vi "BS navigation demo.vi"() -> ()   [LabVIEW 2012]
uses:
  <vilib>/vision/NI_Vision_Development_Module.lvlib
panel:
  out "tug location string":string
  out "All found?":bool
  out "Tug location array":T1(array[cluster])
  in  "Image file name":string="boats and buoys.bmp"
  in  "stop":bool
  out "error out":errorcluster
  out "Working Image":T2(plugin-control)
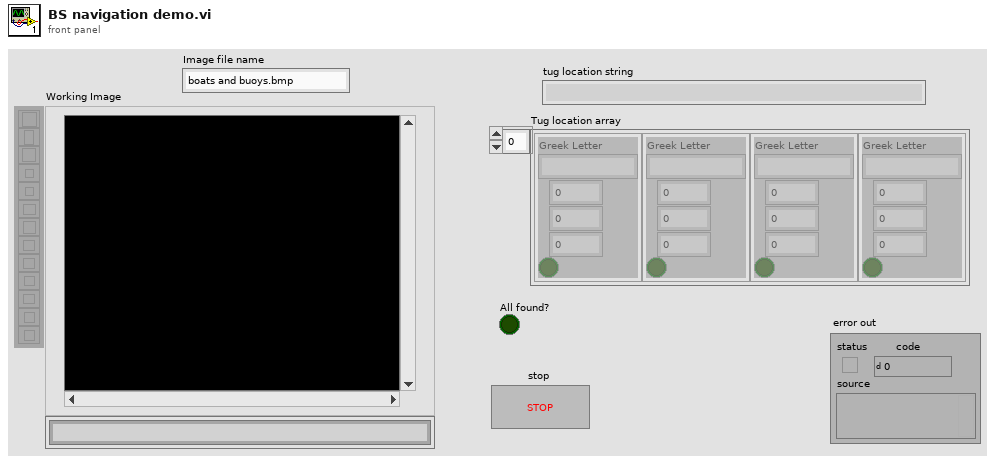
[diagram p1: front panel]
types:
  T1 = cluster{"Greek Letter":string, i16, i16, i16, bool}[]
  T2 = typedef "IMAQ Image.ctl" = refnum<image>
  T3 = typedef "Image Type" = u32
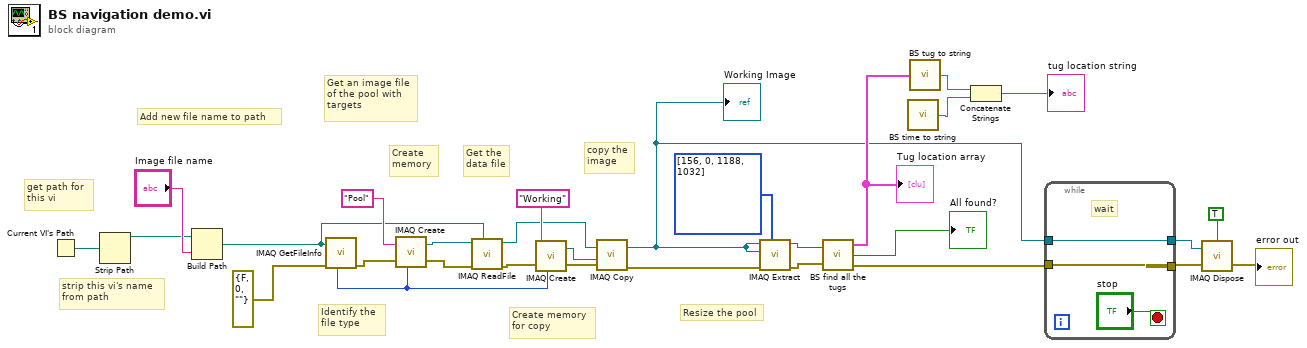
[diagram p0: block diagram]
diagram:
  # "Resize the pool"
  # "Create memory\nfor copy"
  # "copy the\nimage"
  # "Add new file name to path"
  # "strip this vi's name \nfrom path"
  # "get path for \nthis vi"
  # "Get the \ndata file"
  # "Create \nmemory"
  # "Identify the \nfile type"
  # "Get an image file\nof the pool with\ntargets"
  n1 = Current VI's Path() -> (path=w21:path)
  n2 = Strip Path(path=w21) -> (stripped path=w20:path)  [unwired: 1 out]
  n3 = Build Path(base path=w20, name or relative path="Image file name") -> (appended path=w19:path)
  n4 = call "IMAQ GetFileInfo"("error in (no error)"=errorcluster {"status"=FALSE, "code"=0, "source"=""}, "File Path"=w19) -> ("error out"=w30:errorcluster, "Image Type"=w12:T3)  [unwired: 3 in, 5 out]
  n5 = call "IMAQ Create"("Image Name"="Pool", "Image Type"=w12, "error in (no error)"=w30) -> ("New Image"=w28:T2, "error out"=w25:errorcluster)  [unwired: 2 in]
  n6 = call "IMAQ ReadFile"("File Path"=w19, "error in (no error)"=w25, "Image"=w28) -> ("error out"=w13:errorcluster, "Image Out"=w14:T2)  [unwired: 4 in, 3 out]
  n7 = call "IMAQ Create"("Image Name"="Working", "Image Type"=w12, "error in (no error)"=w13) -> ("New Image"=w23:T2, "error out"=w26:errorcluster)  [unwired: 2 in]
  n8 = call "IMAQ Copy"("error in (no error)"=w26, "Image Dst"=w23, "Image Src"=w14) -> ("error out"=w7:errorcluster, "Image Dst Out"=w6:T2)  [unwired: 3 in]
  "Working Image" <- w6
  n9 = call "IMAQ Extract"("Optional Rectangle"=i32[] [156, 0, 1188, 1032], "error in (no error)"=w7, "Image Dst"=w6, "Image Src"=w6) -> ("error out"=w5:errorcluster, "Image Dst Out"=w4:T2)  [unwired: 6 in]
  n10 = call "BS find all the tugs.vi"("Image Src"=w4, "error in"=w5) -> ("Tug location array"=w9:T1, "All found?"=→"All found?":bool, "error out"=w11:errorcluster)
  "Tug location array" <- w9
  n11 = call "BS time to string.vi"() -> ("time string"=w2:string)  [unwired: 1 in]
  n12 = call "BS tug to string.vi"("Tug location array"=w9) -> ("tug location string"=w3:string)
  n13 = Concatenate Strings(w3, w2) -> (→"tug location string":string)
  n14 = while {
    tunnel: w6 -> [w31]
    tunnel: w11 -> [w32]
    tunnel: [w32] -> w18
    tunnel: [w31] -> w16
    stop <- "stop" stop-if-true
    # "wait"
  }
  n15 = call "IMAQ Dispose"("All Images? (No)"=TRUE, "Image"=w16, "error in (no error)"=w18) -> ("error out"=→"error out":errorcluster)  [unwired: 3 in]
